vi "PH_PPPA_PowerUnit.calc Status.vi"(0 "i ref in":refnum<vi>, 5 "error in (no error)":errorcluster) -> (14 "i ref out":refnum<vi>, 19 "error out":errorcluster)   [LabVIEW 2014, in "PH_PPPA_PowerUnit.lvlib"]
doc: "This VI checks wether one of the subsystems is in failure or alarm status, if there is no information about the system or whether systems are off. It writes the information to own attributes, the GUI and publishes it as DIM service."
uses:
  PH_PPPA_PowerUnit.lvlib
  PH_Basics/PH_StatusHandler/PH_StatusHandler.Status.ctl
  PH_Basics/PH_SystemInformation/PH_SystemInformationEnabling State.ctl
  PH_Basics/PH_StatusHandler/PH_StatusHandler.lvlib
  PH_Basics/PH_SystemInformation/PH_SystemInformation.lvlib
  PH_Basics/PH_PowerUnit_BaseClass/PH_PowerUnit_BaseClass.lvlib
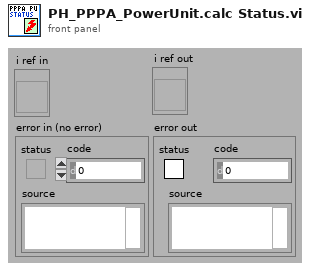
[diagram p1: front panel]
types:
  T1 = typedef "PH_StatusHandler.lvlib/PH_StatusHandler.Status.ctl" = i16
  T2 = typedef "PH_PPPA_PowerUnit.lvlib/PH_PPPA_PowerUnit.i attribute.ctl" = cluster{"GUI Refs":cluster{"Ignitron":refnum<vi>, "Rossrelais":refnum<vi>, "Set Voltage":refnum<vi>, "PSU":refnum<vi>, "EOC":refnum<vi>, "Trigger":refnum<vi>}, "Ignitron":T3, "PSU":T4, "Dump Ross Relais":T5, "Trigger":cluster{"State Device":T1, "linked?":bool}, "Timing Settings":cluster{"Prdc Fast?":bool, "Default Value Periodic Interval":i32, "Mercury on since":dbl, "Warm up Time Mercury [s]":dbl}, "Set Voltage [V]":dbl, "19er Ignitionbox":string}
  T3 = typedef "PH_PP_Common.lvlib/PH_PP_Common.Ignitron Attributes.ctl" = cluster{"State Device":T1, "linked?":bool}
  T4 = typedef "PH_PP_Common.lvlib/PH_PP_Common.PSU Attributes.ctl" = cluster{"lower limit [V]":dbl, "upper limit [V]":dbl, "Voltage set":bool, "State Device":T1, "linked?":bool}
  T5 = typedef "PH_PP_Common.lvlib/PH_PP_Common.Ross Relais Attributes.ctl" = cluster{"State Device":T1, "linked?":bool}
  T6 = typedef "PH_PowerUnit_BaseClass.lvlib/PH_PowerUnit_BaseClass.i attribute.ctl" = cluster{"Constructor finished":bool, "PU":cluster{"In use":bool, "Service ID in use":i32, "GUI Ref":refnum<vi>}, "Enabling":cluster{"State":T7, "GUI Ref":refnum<vi>}, "Timing":cluster{"Last Shot":dbl, "Time between Shots [Sec]":dbl, "Waiting Time over?":bool, "Service ID Waiting Time":i32, "GUI Ref":refnum<vi>, "Instance":cluster{"Status":T1, "linked?":bool, "GUI Ref":refnum<vi>}}, "Sequencer":cluster{"SM State":string, "GUI Ref":refnum<vi>, "linked":bool}, "Subscribed Trendmssgs":cluster{"Tagname":string, "Status":T1, "linked?":bool, "Shot Condition":T1, "GUI Ref":refnum<vi>}[], "PP PU":T8, "Default Voltage (V)":dbl, "GUI Refs":T9, "PSDB data":cluster{"Shot Voltage [V]":dbl, "State TO SM":T10, "Write 2 early":bool}, "State TO SM":T10}
  T7 = typedef "PH_SystemInformation.lvlib/PH_SystemInformationEnabling State.ctl" = i32
  T8 = typedef "PH_PP_Common.lvlib/PH_PP_Common.PUs.ctl" = enum16{"no Info", "PA-19mm-1", "PA-19mm-2", "PA-45mm-PILC", "PA-45mm-MAIN", "MA-PU-1", "MA-PU-2", "MA-PU-3", "MA-PU-4", "MA-PU-5", "MA-PU-6", "MA-FR", "MA-PILC", "PA-45mm-DP"}
  T9 = typedef "PH_PowerUnit_BaseClass.lvlib/PH_PowerUnit_BaseClass.GUI Refs.ctl" = cluster{"Delete Inst":refnum<vi>, "State TO SM":refnum<vi>, "State SM":refnum<vi>, "Fire":refnum<vi>}
  T10 = typedef "PH_PowerUnit_BaseClass.lvlib/PH_PowerUnit_BaseClass.SM States.ctl" = enum16{".", "Stand by", "Switch PU on", "Configure", "Set Default Voltage", "Set STANDBY", "Set READY", "Wait for Shot Cmd", "Open Dump Rods", "Open Ross Relais", "Close Ross Relais", "Switch PSU on", "Switch PSU off", "Charge", "Switch GD Channel on", "Close Dump Rods", "Rods-TO", "RR-TO", "PSU-TO", "Trigger-TO"}
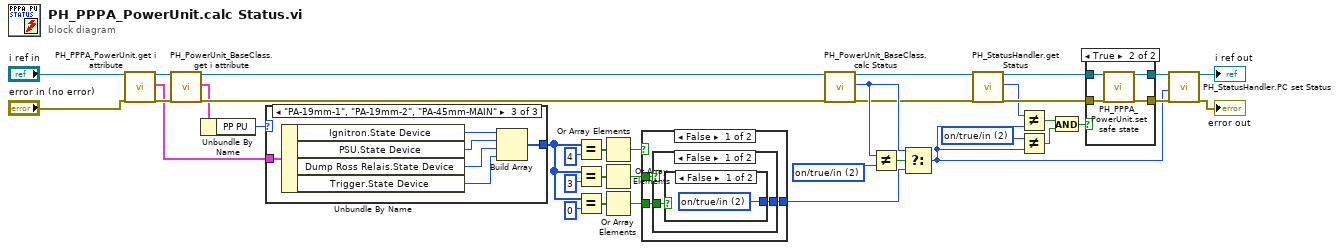
[diagram p0: block diagram]
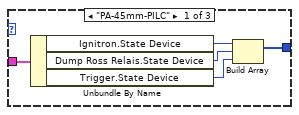
[diagram p2: hidden frame]
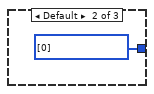
[diagram p3: hidden frame]
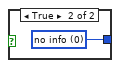
[diagram p4: hidden frame]
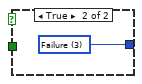
[diagram p5: hidden frame]
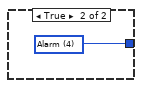
[diagram p6: hidden frame]
diagram:
  w16 = T1 2 items=["no info", "off/false/out", "on/true/in", "Failure", "Alarm", "Status 1", "Status 2", "Status 3"] ("Device Status")
  w19 = T1 2 items=["no info", "off/false/out", "on/true/in", "Failure", "Alarm", "Status 1", "Status 2", "Status 3"] ("y")
  n1 = call "PH_PPPA_PowerUnit.get i attribute.vi"("i ref in"="i ref in", "error in (no error)"="error in (no error)") -> ("i ref out"=w25:refnum<vi>, "i attribute"=w8:T2, "error out"=w28:errorcluster)  [unwired: 15 in]
  n2 = call "PH_PowerUnit_BaseClass.get i attribute.vi"("i ref in"=w25, "error in (no error)"=w28) -> ("i ref out"=w14:refnum<vi>, "i attribute"=w7:T6, "error out"=w13:errorcluster)  [unwired: 15 in]
  n3 = Unbundle By Name(w7) -> ("PP PU"=w6:T8)
  n4 = case shown="\"PA-19mm-1\", \"PA-19mm-2\", \"PA-45mm-MAIN\"" w6 {
    tunnel: [w39 w43 w46] -> w9
    tunnel: w8 -> [w38 _ w45]
    frame "PA-45mm-PILC" {
      n5 = Unbundle By Name(w38) -> ("Ignitron.State Device"=w42:T1, "Dump Ross Relais.State Device"=w41:T1, "Trigger.State Device"=w40:T1)
      n6 = Build Array(w42, w41, w40) -> (w39:T1[])
    }
    frame Default {
      w43 = T7[] [0] items=["no info", "not disabled", "disabled"]
    }
    frame "PA-19mm-1", "PA-19mm-2", "PA-45mm-MAIN" {
      n7 = Unbundle By Name(w45) -> ("Ignitron.State Device"=w44:T1, "PSU.State Device"=w49:T1, "Dump Ross Relais.State Device"=w48:T1, "Trigger.State Device"=w47:T1)
      n8 = Build Array(w44, w49, w48, w47) -> (w46:T1[])
    }
  }
  n9 = Equal?(x=w9, y=4) -> (x = y?=w36:bool[])
  n10 = Equal?(x=w9, y=3) -> (x = y?=w34:bool[])
  n11 = Equal?(x=w9, y=0) -> (x = y?=w32:bool[])
  n12 = Or Array Elements(Boolean array=w36) -> (logical OR=w31:bool)
  n13 = Or Array Elements(Boolean array=w34) -> (logical OR=w30:bool)
  n14 = Or Array Elements(Boolean array=w32) -> (logical OR=w29:bool)
  n15 = case shown="False" w31 {
    tunnel: [w52 w58] -> w10
    tunnel: w30 -> [w51 _]
    tunnel: w29 -> [w50 _]
    frame False {
      n16 = case shown="False" w51 {
        tunnel: [w54 w57] -> w52
        tunnel: w50 -> [w53 _]
        frame False {
          n17 = case shown="False" w53 {
            tunnel: [w55 w56] -> w54
            frame False {
              w55 = T1 2 items=["no info", "off/false/out", "on/true/in", "Failure", "Alarm", "Status 1", "Status 2", "Status 3"] ("Device Status")
            }
            frame True {
              w56 = T1 0 items=["no info", "off/false/out", "on/true/in", "Failure", "Alarm", "Status 1", "Status 2", "Status 3"] ("Device Status")
            }
          }
        }
        frame True {
          w57 = T1 3 items=["no info", "off/false/out", "on/true/in", "Failure", "Alarm", "Status 1", "Status 2", "Status 3"] ("Device Status")
        }
      }
    }
    frame True {
      w58 = T1 4 items=["no info", "off/false/out", "on/true/in", "Failure", "Alarm", "Status 1", "Status 2", "Status 3"] ("Device Status")
    }
  }
  n18 = call "PH_PowerUnit_BaseClass.calc Status.vi"("VI in"=w14, "error in (no error)"=w13) -> ("VI out"=w3:refnum<vi>, "PU Status"=w18:T1, "error out"=w5:errorcluster)  [unwired: 15 in]
  n19 = Not Equal?(x=w18, y=w19) -> (x != y?=w20:bool)
  n20 = Select(t=w18, s=w20, f=w10) -> (s? t:f=w11:T1)
  n21 = call "PH_StatusHandler.get Status.vi"("VI in"=w3, "error in"=w5) -> ("VI out"=w2:refnum<vi>, "Status"=w1:T1, "error out"=w4:errorcluster)  [unwired: 15 in]
  n22 = Not Equal?(x=w1, y=w11) -> (x != y?=w17:bool)
  n23 = Not Equal?(x=w16, y=w11) -> (x != y?=w15:bool)
  n24 = And(x=w17, y=w15) -> (x .and. y?=w12:bool)
  n25 = case shown="True" w12 {
    tunnel: w2 -> [w60 w64]
    tunnel: w4 -> [w59 w63]
    tunnel: [w60 w62] -> w24
    tunnel: [w59 w61] -> w22
    frame False {
    }
    frame True {
      n26 = call "PH_PPPA_PowerUnit.set safe state.vi"("i ref in"=w64, "error in (no error)"=w63) -> ("i ref out"=w62:refnum<vi>, "error out"=w61:errorcluster)  [unwired: 16 in]
    }
  }
  n27 = call "PH_StatusHandler.PC set Status.vi"("i ref in"=w24, "Status"=w11, "error in (no error)"=w22) -> ("i ref out"=→"i ref out":refnum<vi>, "error out"=→"error out":errorcluster)  [unwired: 15 in]
